vi "Measurement Parser.vi"(7 "Waveform Graph":dynamicdata(graph), 8 "error in (no error)":errorcluster, 9 "Generic Card in":refnum<class "Generic Card.lvclass">, 10 "Data Array":dbl[](array[numeric]), 11 "Generic Digital Multi Meter in":refnum<class "Generic Digital Multi Meter.lvclass">) -> (0 "error out":errorcluster, 3 "Generic Digital Multi Meter out":refnum<class "Generic Digital Multi Meter.lvclass">)   [LabVIEW 2014, in "Generic Digital Multi Meter.lvlib" / "Generic Digital Multi Meter.lvclass"]
uses:
  Generic Digital Multi Meter.lvclass
  Generic Instrument/Generic Card/Generic Card.lvclass
  Abstract Sensor/Abstract Sensor.lvclass
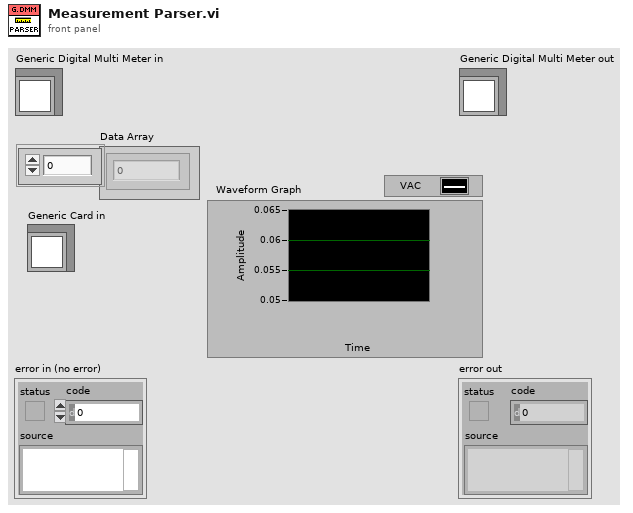
[diagram p1: front panel]
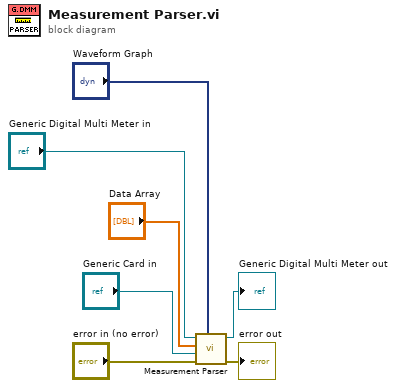
[diagram p0: block diagram]
diagram:
  n1 = call-parent "Measurement Parser.vi"("Waveform Graph"="Waveform Graph", "error in (no error)"="error in (no error)", "Generic Card in"="Generic Card in", "Data Array"="Data Array", "Abstract Sensor in"="Generic Digital Multi Meter in") -> ("error out"=→"error out":errorcluster, "Abstract Sensor out"=→"Generic Digital Multi Meter out":refnum<class "Generic Digital Multi Meter.lvclass">)  [unwired: 5 in]
